vi "chip_erase_new_Flash.vi"(2 "write array":u8[](array[numeric]) format="%x") -> ()   [LabVIEW 2022 SP3]
panel:
  out "InputReport1":u8[](array[numeric]) format="%x"
  out "Output Report":u8[](array[numeric])
  out "Input Report":u8[](array[numeric])
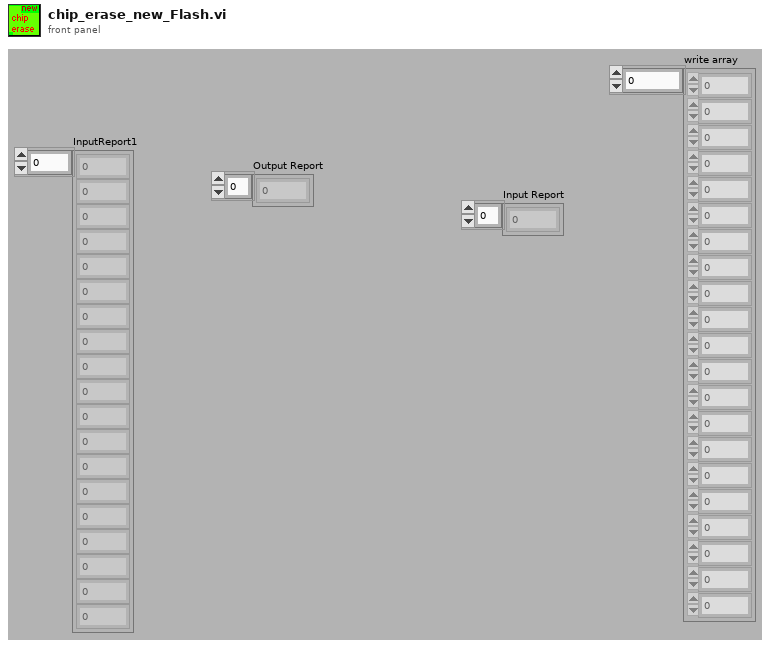
[diagram p1: front panel]
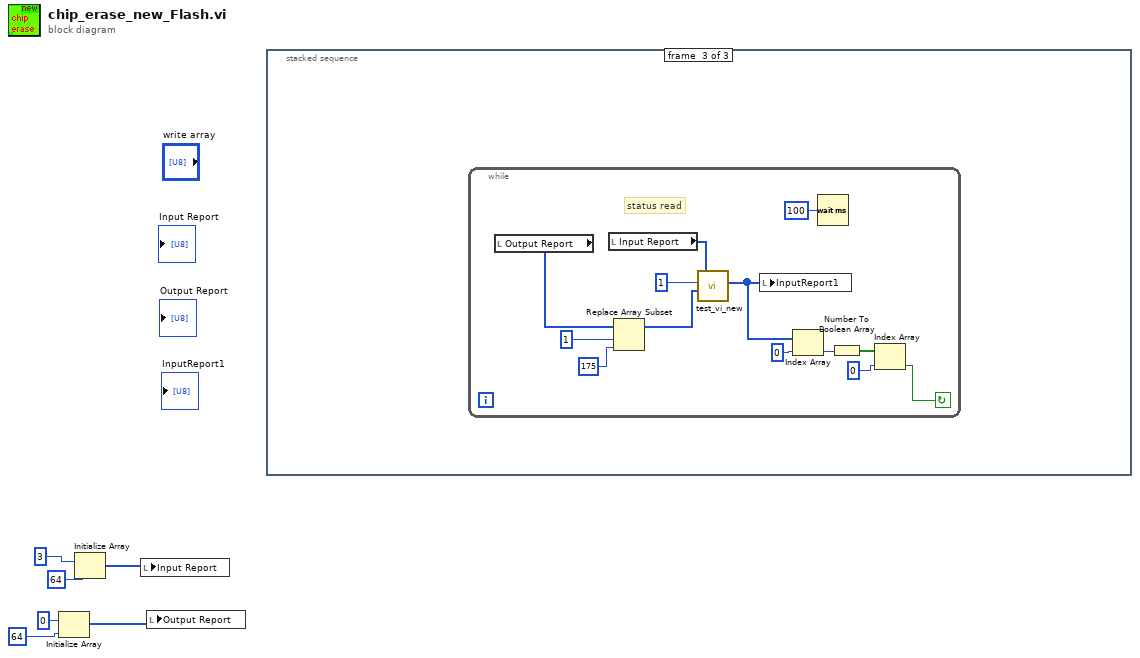
[diagram p0: block diagram]
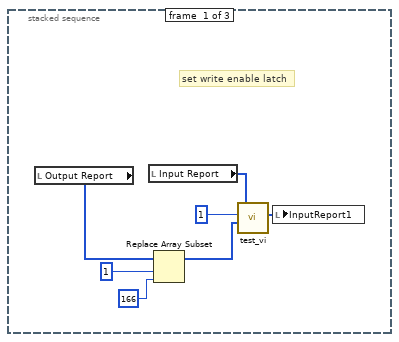
[diagram p2: hidden frame]
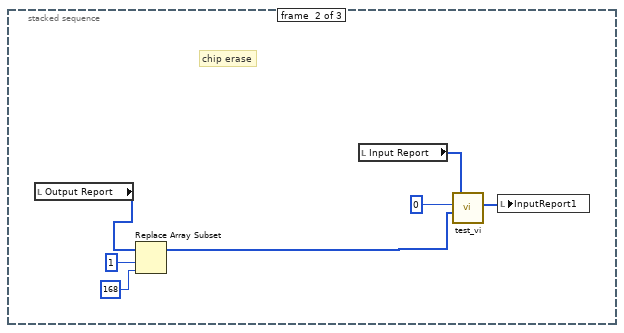
[diagram p3: hidden frame]
diagram:
  n1 = Initialize Array(u8 0 ("element"), 64 ("dimension size")) -> (w1:u8[])
  n2 = Initialize Array(u8 3 ("element"), 64 ("dimension size")) -> (w2:u8[])
  n3 = local write "Input Report"(w2) -> ()
  n4 = local write "Output Report"(w1) -> ()
  n5 = stacked-sequence {
    frame #0 {
      # "set write enable latch"
      n6 = local read "Output Report"() -> (w10:u8[])
      n7 = local read "Input Report"() -> (w9:u8[])
      n8 = Replace Array Subset(array=w10, new element=u8 166 ("new element/subarray"), index=1) -> (w8:u8[])
      n9 = call "test_vi.vi"("OutputReport_in"=w8, "DevDet_in"=1, "InputReport_in"=w9) -> ("InputReport_out"=w7:u8[])  [unwired: 1 in, 3 out]
      n10 = local write "InputReport1"(w7) -> ()
    }
    frame #1 {
      # "chip erase"
      n11 = local read "Output Report"() -> (w17:u8[])
      n12 = Replace Array Subset(array=w17, new element=u8 168 ("new element/subarray"), index=1) -> (w14:u8[])
      n13 = local read "Input Report"() -> (w16:u8[])
      n14 = call "test_vi.vi"("OutputReport_in"=w14, "DevDet_in"=0, "InputReport_in"=w16) -> ("InputReport_out"=w15:u8[])  [unwired: 1 in, 3 out]
      n15 = local write "InputReport1"(w15) -> ()
    }
    frame #2 {
      n16 = while {
        stop <- w22 continue-if-true
        # "status read"
        n17 = local read "Output Report"() -> (w30:u8[])
        n18 = local read "Input Report"() -> (w29:u8[])
        n19 = Replace Array Subset(array=w30, new element=u8 175 ("new element/subarray"), index=1) -> (w28:u8[])
        n20 = call "test_vi_new.vi"("OutputReport_in"=w28, "DevDet_in"=1, "InputReport_in"=w29) -> ("InputReport_out"=w23:u8[])  [unwired: 1 in, 3 out]
        n21 = local write "InputReport1"(w23) -> ()
        n22 = Index Array(array=w23, index=0) -> (element=w26:u8)
        n23 = Wait (ms)(milliseconds to wait=u32 100) -> ()  [unwired: 1 out]
        n24 = Number To Boolean Array(number=w26) -> (Boolean array=w25:bool[])
        n25 = Index Array(array=w25, index=0) -> (element=w22:bool)
      }
    }
  }
